vi "Motor_Plus_Impedance_controller.14_07_2017_4vi.vi"() -> ()   [LabVIEW 2016]
uses:
  <vilib>/Motion/Express/_s/nimc.fb.stopMove.stop.axis.modeDecelerate.vi
  <vilib>/Motion/Express/_s/nimc.fb.read.readExecutionData.axis.vi
  <vilib>/Motion/Express/_s/nimc.fb.straightLineMove.startStraightLineMove.axis.modeVelocity.0.vi
  <vilib>/Motion/PropertyNodes/nimc.createStraightLineMoveInstance.axis.vi
  <vilib>/Motion/Express/_s/nimc.ax.power.power.axis.vi
  <vilib>/Motion/BlockNode/FB.NIMotion.xnode
panel:
  in  "Enable Axis \nControl 2":bool
  in  "Numeric":i32=2
  in  "Move to Position?":bool
  out "Torque":dbl(knob) scale=0.0..10.0
  out "Position":dbl(knob) scale=0.0..10.0
  out "Velocity":dbl(knob) scale=0.0..10.0
  out "Load Cell":dbl(knob) scale=0.0..10.0
  in  "desired motor\nposition":dbl
  out "Load cell, V":dbl format="%.3f"
  out "motor torque, Nm":dbl format="%.3f"
  out "motor velocity, rev/s":dbl format="%.3f"
  out "motor position, rev":dbl format="%.3f"
  in  "STOP VI":bool
  in  "Enable Axis \nControl":bool
  in  "Enable Motor \nDrive":bool
  in  "EMERGENCY MOTOR STOP":bool
  # "Raw Data from System"
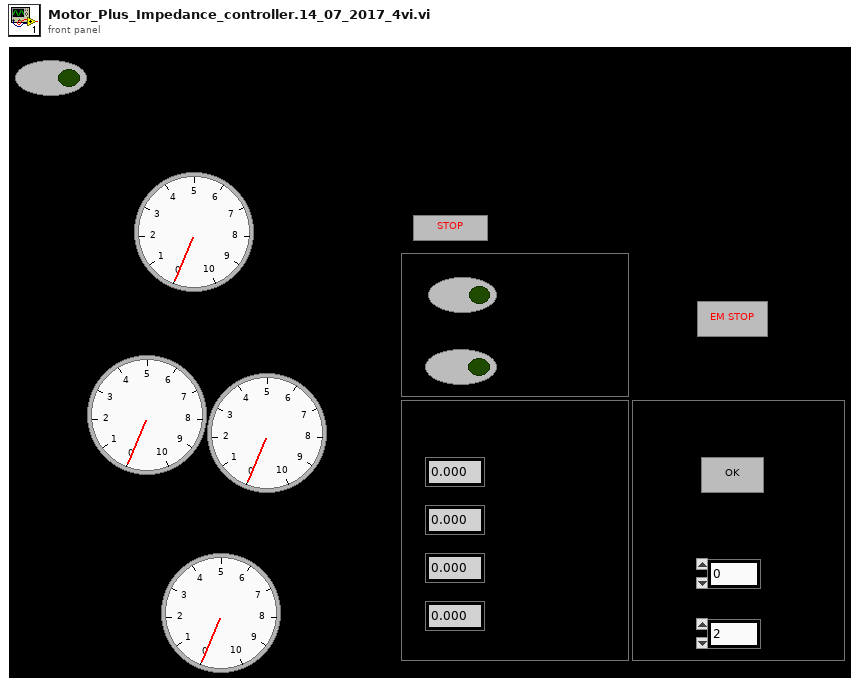
[diagram p1: front panel]
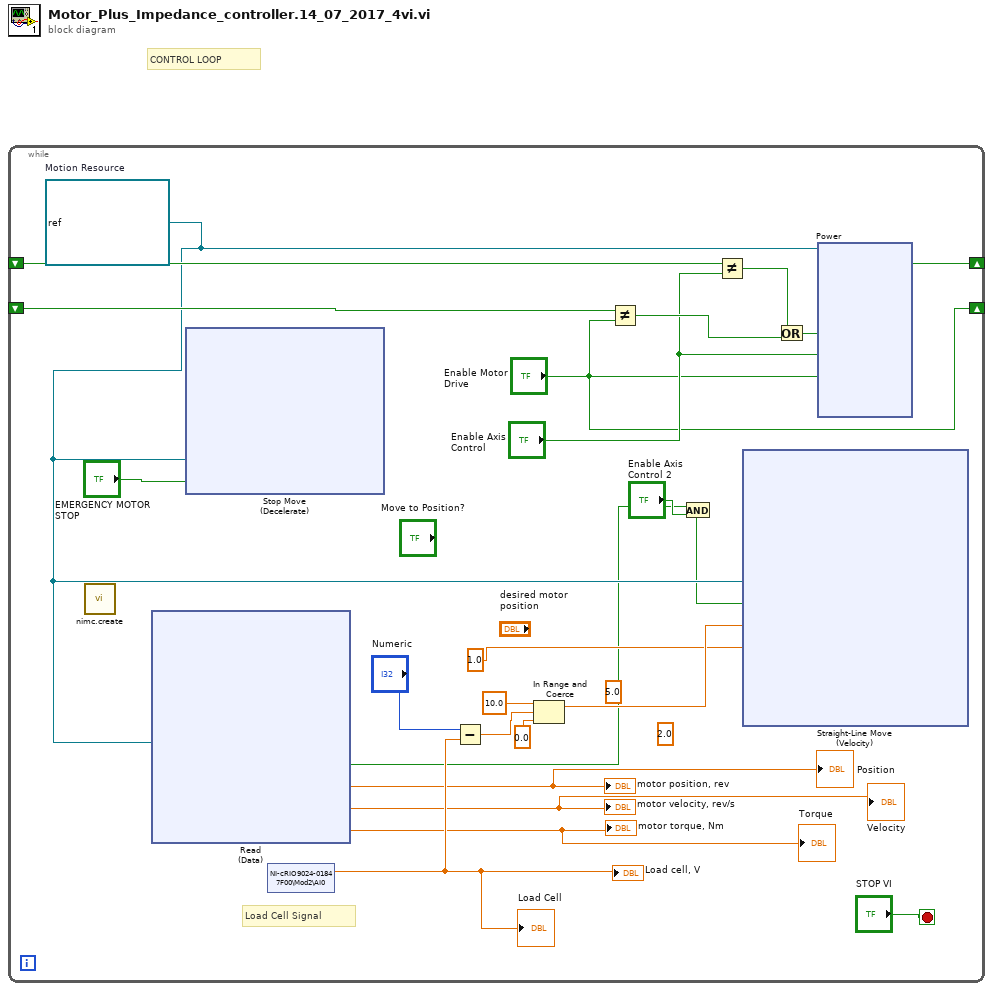
[diagram p0: block diagram]
diagram:
  # "CONTROL LOOP"
  n1 = while {
    shift-right: ["Enable Axis \nControl"] -> _
    shift-left: _ -> [w22]
    shift-right: ["Enable Motor \nDrive"] -> _
    shift-left: _ -> [w21]
    stop <- "STOP VI" stop-if-true
    w4 = refnum<k21> "nism://NI-cRIO9024-01847F00/Axis 1"  # Motion Resource
    (unwired) 5.0
    (unwired) 2.0
    # "Load Cell Signal"
    n2 = call-poly <vilib>:"nimc.create.vi"() -> ()  [unwired: 9 in, 3 out]
    n3 = xnode "Read\n(Data)"("resource"=w4) -> ("is valid"=w2:bool, "torque"=→"motor torque, Nm" →"Torque":dbl, "velocity"=→"motor velocity, rev/s" →"Velocity":dbl, "position"=→"motor position, rev" →"Position":dbl)  [unwired: 1 in, 2 out]
    n4 = xnode "Stop Move\n(Decelerate)"("resource"=w4, "execute"="EMERGENCY MOTOR STOP") -> ()  [unwired: 1 in, 3 out]
    n5 = shared-variable "NI-cRIO9024-01847F00\\Mod2\\AI0"() -> (w10:dbl)  [unwired: 1 in, 1 out]
    "Load cell, V" <- w10
    "Load Cell" <- w10
    n6 = Subtract(x="Numeric", y=w10) -> (x-y=w11:dbl)
    n7 = In Range and Coerce(upper limit=10.0, x=w11, lower limit=0.0) -> (coerced(x)=w6:dbl)  [unwired: 1 out]
    n8 = Not Equal?(x=w21, y="Enable Motor \nDrive") -> (x != y?=w19:bool)
    n9 = And(x=w2, y="Enable Axis \nControl 2") -> (x .and. y?=w1:bool)
    n10 = Not Equal?(x=w22, y="Enable Axis \nControl") -> (x != y?=w20:bool)
    n11 = xnode "Straight-Line Move\n(Velocity)"("resource"=w4, "execute"=w1, "velocity"=w6, "acceleration"=1.0) -> ()  [unwired: 1 in, 3 out]
    n12 = Or(x=w20, y=w19) -> (x .or. y?=w18:bool)
    n13 = xnode ("Power")("execute"=w18, "enable axis"="Enable Axis \nControl", "enable drive"="Enable Motor \nDrive", "resource"=w4) -> ()  [unwired: 1 in, 6 out]
  }
